vi "插入testdata并获取id.vi"(4 "Ref":bool=TRUE, 6 "测试类型":u16(ring) items=["直通测试", "校准测试", "电缆"], 7 "数据类型":string="MLOG", 8 "error in (no error)":errorcluster, 9 "出口":i32, 10 "进口":i32, 11 "network in":refnum<class "network.lvclass">) -> (0 "error out":errorcluster, 2 "id":i32, 3 "network out":refnum<class "network.lvclass">)   [LabVIEW 2015]
uses:
  network analyzer/network/network.lvclass
  Ctl/database_Method.ctl
  Ctl/DNS.ctl
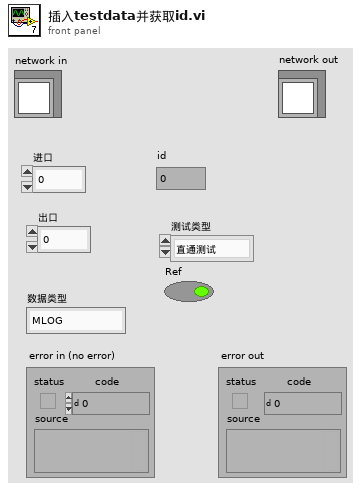
[diagram p1: front panel]
types:
  T1 = typedef "database_Method.ctl" = enum16{"初始化", "查询", "关闭"}
  T2 = typedef "DNS.ctl" = string
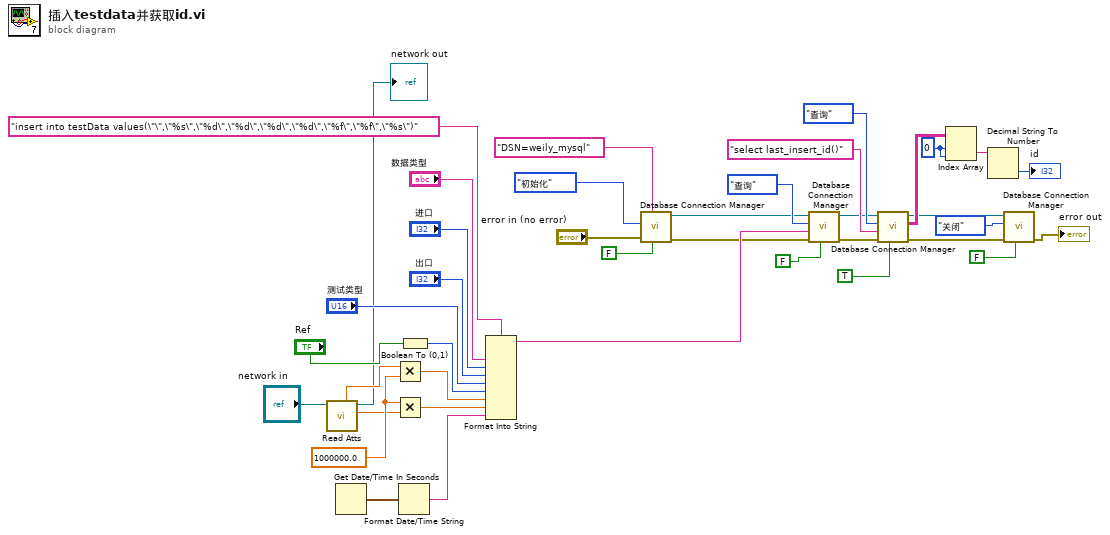
[diagram p0: block diagram]
diagram:
  w17 = 0 ("index (row)")
  w32 = 1000000.0 ("y")
  n1 = call-dynamic "Read Atts.vi"("network in"="network in") -> ("Stop"=w25:dbl, "network out"=→"network out":refnum<class "network.lvclass">, "Start"=w26:dbl)  [unwired: 5 in, 3 out]
  n2 = Get Date/Time In Seconds() -> (seconds since 1Jan1904=w31:timestamp)
  n3 = Multiply(x=w26, y=w32) -> (x*y=w34:dbl)
  n4 = Multiply(x=w32, y=w25) -> (x*y=w35:dbl)
  n5 = Format Date/Time String(seconds (now)=w31) -> (date/time string=w30:string)  [unwired: 2 in]
  n6 = Boolean To (0,1)(Boolean="Ref") -> (0, 1=w38:i16)
  n7 = Format Into String(format string="insert into testData values(\"\",\"%s\",\"%d\",\"%d\",\"%d\",\"%d\",\"%f\",\"%f\",\"%s\")" ("SQL"), "数据类型", "进口", "出口", "测试类型", w38, w34, w35, w30) -> (resulting string=w29:string)  [unwired: 2 in, 1 out]
  n8 = call "Database Connection Manager.vi"("Return Data (T)"=FALSE, "ConnectionString"=T2 "DSN=weily_mysql", "error in (no error)"="error in (no error)", "Method"=database_Method."初始化") -> ("error out"=w6:errorcluster, "ADODB._Connection Out"=w9:refnum<k7>)  [unwired: 4 in, 2 out]
  n9 = call "Database Connection Manager.vi"("Return Data (T)"=FALSE, "error in (no error)"=w6, "Command Text"=w29, "Method"=database_Method."查询", "ADODB._Connection In"=w9) -> ("error out"=w21:errorcluster, "ADODB._Connection Out"=w8:refnum<k7>)  [unwired: 3 in, 2 out]
  n10 = call "Database Connection Manager.vi"("Return Data (T)"=TRUE, "error in (no error)"=w21, "Command Text"="select last_insert_id()", "Method"=database_Method."查询", "ADODB._Connection In"=w8) -> ("error out"=w2:errorcluster, "Data"=w15:string[][], "ADODB._Connection Out"=w1:refnum<k7>)  [unwired: 3 in, 1 out]
  n11 = Index Array(array=w15, index (row)=w17, index (col)=w17) -> (element=w16:string)
  n12 = Decimal String To Number(string=w16) -> (number=→"id":i32)  [unwired: 2 in, 1 out]
  n13 = call "Database Connection Manager.vi"("Return Data (T)"=FALSE, "error in (no error)"=w2, "Method"=database_Method."关闭", "ADODB._Connection In"=w1) -> ("error out"=→"error out":errorcluster)  [unwired: 4 in, 3 out]
